vi "ZC_hetong.vi"(0 "action":string, 1 "LabVIEW Web Service Request":refnum<class "Web Request.lvclass"> caption="LabVIEW Web服务请求", 2 "fpbh":string, 3 "gmjg":string, 5 "id":string, 6 "key":string, 7 "name":string, 8 "number":string, 9 "bianhao":string, 10 "shuliang":string, 11 "gysh":string, 12 "gmriqi":string, 13 "bxnx":string, 14 "beizhu":string, 15 "gmzc":string) -> (4 "error":errorcluster)   [LabVIEW 2017]
uses:
  <vilib>/wsapi/Web Request.lvclass
panel:
  out "postdata":string caption="post数据"
  out "error out":errorcluster caption="错误输出"
  # "Web服务请求输入接线端用于调用“Web服务”选板的VI。除非不需要访问该选板，否则不要在连线板上删除这个输入接线端。"
  # "添加至连线板的每一个其他输入控件，在URL中对应于一个输入。如需在接线端模式输出（默认设置）下包含显示控件，则该显示控件必须与连线板相连。"
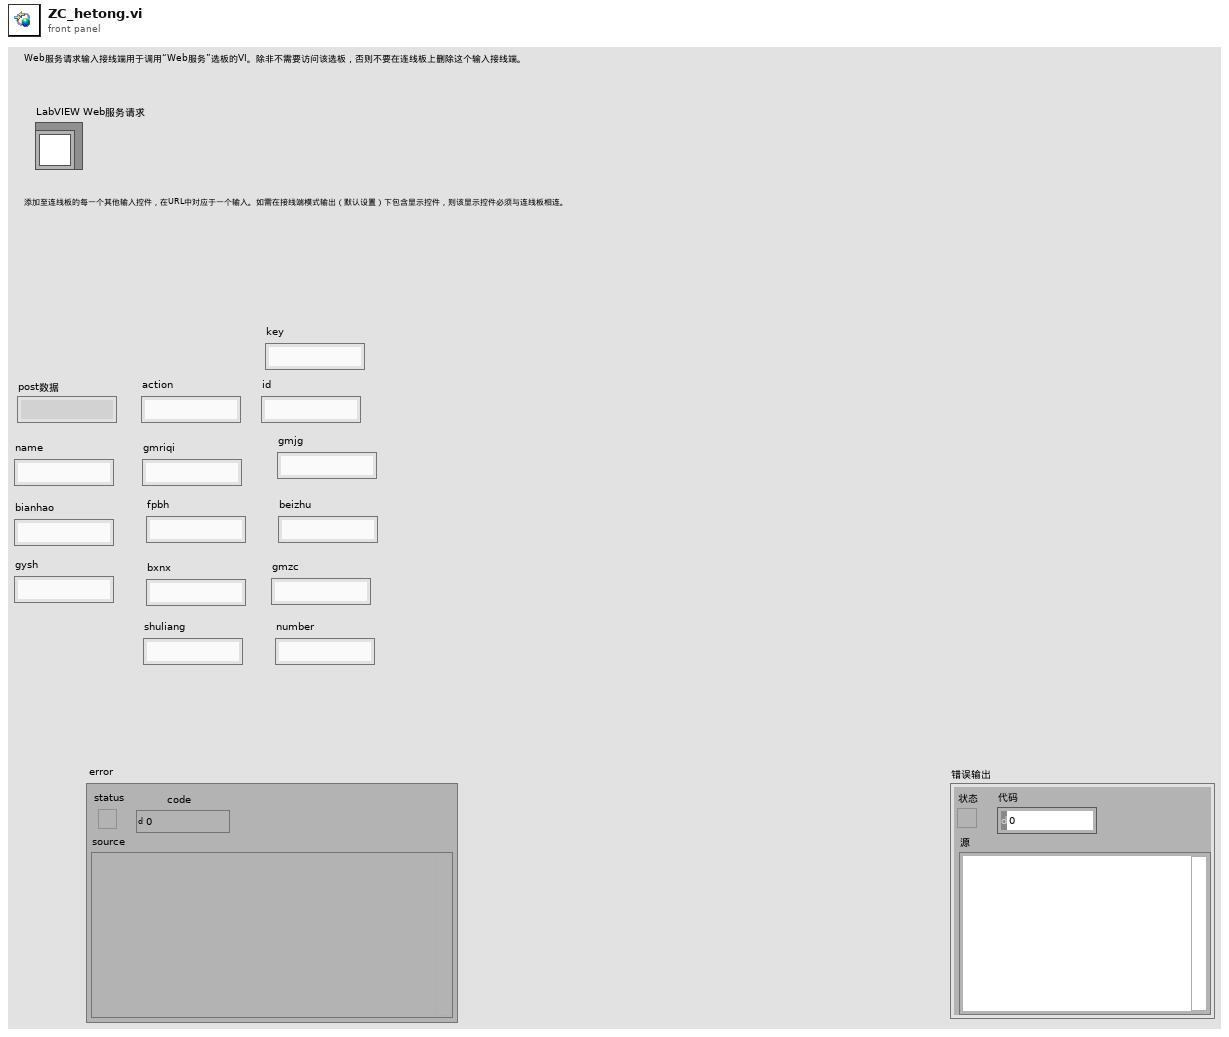
[diagram p1: front panel]
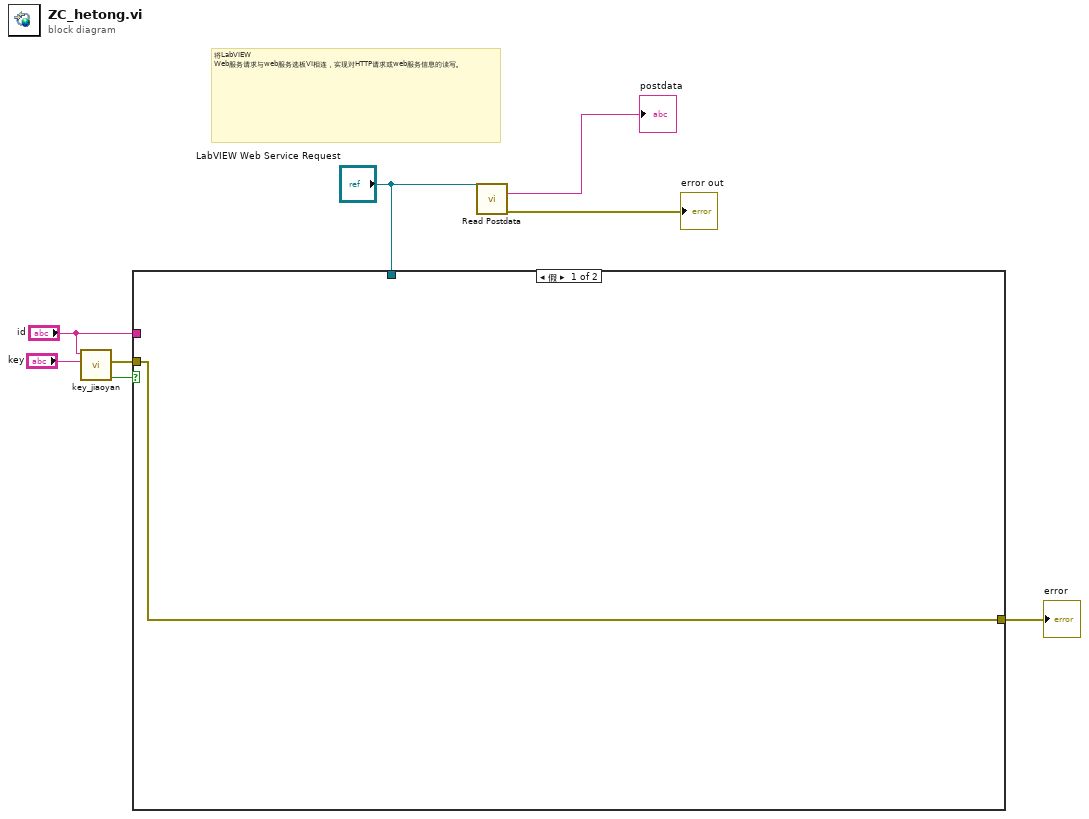
[diagram p0: block diagram]
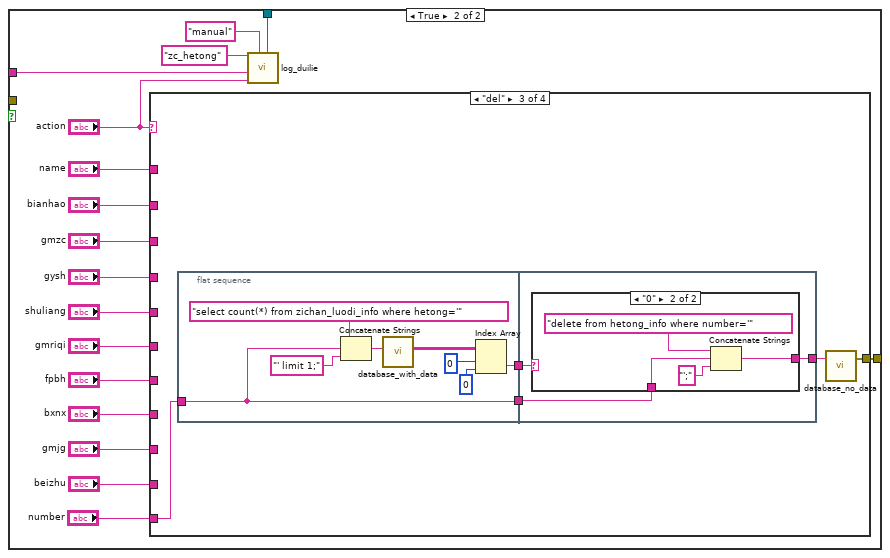
[diagram p2: hidden frame]
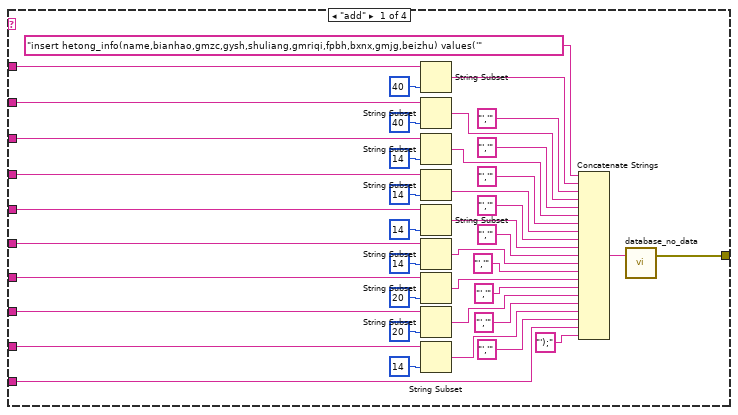
[diagram p3: hidden frame]
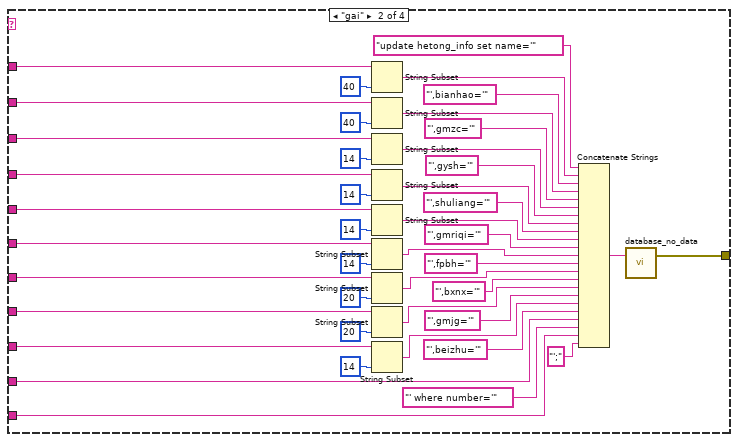
[diagram p4: hidden frame]
diagram:
  # "将LabVIEW Web服务请求与web服务选板VI相连，实现对HTTP请求或web服务信息的读写。"
  n1 = call "key_jiaoyan.vi"("key_client"="key", "gonghao"="id") -> ("jy"=w2:bool, "error"=w1:errorcluster)  [unwired: 8 in]
  n2 = case shown="假" w2 {
    tunnel: [w9 w15] -> w7
    tunnel: "LabVIEW Web Service Request" -> [_ w12]
    tunnel: "id" -> [_ w10]
    tunnel: w1 -> [w9 _]
    frame False {
    }
    frame True {
      n3 = case shown="\"del\"" "action" {
        tunnel: [w37 w85 w111 _] -> w15
        tunnel: "shuliang" -> [w36 w84 _ _]
        tunnel: "gmzc" -> [w35 w83 _ _]
        tunnel: "gmjg" -> [w34 w82 _ _]
        tunnel: "beizhu" -> [w33 w81 _ _]
        tunnel: "bxnx" -> [w32 w80 _ _]
        tunnel: "fpbh" -> [w31 w79 _ _]
        tunnel: "gmriqi" -> [w30 w78 _ _]
        tunnel: "gysh" -> [w29 w77 _ _]
        tunnel: "bianhao" -> [w28 w76 _ _]
        tunnel: "name" -> [w27 w75 _ _]
        tunnel: "number" -> [_ w70 w112 _]
        frame "add" {
          n4 = String Subset(string=w27, length (rest)=40 ("长度（剩余）")) -> (substring=w63:string)  [unwired: 1 in]
          n5 = String Subset(string=w28, length (rest)=40 ("长度（剩余）")) -> (substring=w61:string)  [unwired: 1 in]
          n6 = String Subset(string=w35, length (rest)=14 ("长度（剩余）")) -> (substring=w43:string)  [unwired: 1 in]
          n7 = String Subset(string=w29, length (rest)=14 ("长度（剩余）")) -> (substring=w59:string)  [unwired: 1 in]
          n8 = String Subset(string=w36, length (rest)=14 ("长度（剩余）")) -> (substring=w39:string)  [unwired: 1 in]
          n9 = String Subset(string=w30, length (rest)=14 ("长度（剩余）")) -> (substring=w57:string)  [unwired: 1 in]
          n10 = String Subset(string=w31, length (rest)=20 ("长度（剩余）")) -> (substring=w52:string)  [unwired: 1 in]
          n11 = String Subset(string=w32, length (rest)=20 ("长度（剩余）")) -> (substring=w49:string)  [unwired: 1 in]
          n12 = String Subset(string=w34, length (rest)=14 ("长度（剩余）")) -> (substring=w46:string)  [unwired: 1 in]
          n13 = Concatenate Strings("insert hetong_info(name,bianhao,gmzc,gysh,shuliang,gmriqi,fpbh,bxnx,gmjg,beizhu) values('" ("格式字符串"), w63, "','" ("字符串"), w61, "','" ("字符串"), w43, "','" ("字符串"), w59, "','" ("字符串"), w39, "','" ("字符串"), w57, "','" ("字符串"), w52, "','" ("字符串"), w49, "','" ("字符串"), w46, "','" ("字符串"), w33, "');" ("字符串")) -> (w38:string)
          n14 = call "database_no_data.vi"("input"=w38) -> ("error"=w37:errorcluster)  [unwired: 2 in]
        }
        frame "gai" {
          n15 = String Subset(string=w75, length (rest)=40 ("长度（剩余）")) -> (substring=w106:string)  [unwired: 1 in]
          n16 = String Subset(string=w76, length (rest)=40 ("长度（剩余）")) -> (substring=w104:string)  [unwired: 1 in]
          n17 = String Subset(string=w83, length (rest)=14 ("长度（剩余）")) -> (substring=w90:string)  [unwired: 1 in]
          n18 = String Subset(string=w77, length (rest)=14 ("长度（剩余）")) -> (substring=w73:string)  [unwired: 1 in]
          n19 = String Subset(string=w84, length (rest)=14 ("长度（剩余）")) -> (substring=w72:string)  [unwired: 1 in]
          n20 = String Subset(string=w78, length (rest)=14 ("长度（剩余）")) -> (substring=w101:string)  [unwired: 1 in]
          n21 = String Subset(string=w79, length (rest)=20 ("长度（剩余）")) -> (substring=w68:string)  [unwired: 1 in]
          n22 = String Subset(string=w80, length (rest)=20 ("长度（剩余）")) -> (substring=w74:string)  [unwired: 1 in]
          n23 = String Subset(string=w82, length (rest)=14 ("长度（剩余）")) -> (substring=w93:string)  [unwired: 1 in]
          n24 = Concatenate Strings("update hetong_info set name='" ("格式字符串"), w106, "',bianhao='" ("字符串"), w104, "',gmzc='" ("字符串"), w90, "',gysh='" ("字符串"), w73, "',shuliang='" ("字符串"), w72, "',gmriqi='" ("字符串"), w101, "',fpbh='" ("字符串"), w68, "',bxnx='" ("字符串"), w74, "',gmjg='" ("字符串"), w93, "',beizhu='" ("字符串"), w81, "' where number='" ("字符串"), w70, "';" ("字符串")) -> (w86:string)
          n25 = call "database_no_data.vi"("input"=w86) -> ("error"=w85:errorcluster)  [unwired: 2 in]
        }
        frame "del" {
          n26 = flat-sequence {
            tunnel: w112 -> [w121]
            tunnel: [w121] -> w115
            tunnel: [w116] -> w114
            tunnel: [w126] -> w113
            tunnel: w115 -> [w125]
            tunnel: w114 -> [w124]
            frame #0 {
              n27 = Concatenate Strings("select count(*) from zichan_luodi_info where hetong='" ("格式字符串"), w121, "' limit 1;" ("字符串")) -> (w120:string)
              n28 = call "database_with_data.vi"("input"=w120) -> ("Data"=w117:string[][])  [unwired: 9 in, 1 out]
              n29 = Index Array(array=w117, index (row)=0 ("索引 (行)"), index (col)=0 ("禁用的索引 (列)")) -> (element=w116:string)
            }
            frame #1 {
              n30 = case shown="\"0\"" w124 {
                tunnel: [_ w128] -> w126
                tunnel: w125 -> [_ w127]
                frame "假", Default {
                }
                frame "0" {
                  n31 = Concatenate Strings("delete from hetong_info where number='" ("格式字符串"), w127, "';" ("字符串")) -> (w128:string)
                }
              }
            }
          }
          n32 = call "database_no_data.vi"("input"=w113) -> ("error"=w111:errorcluster)  [unwired: 2 in]
        }
        frame Default {
        }
      }
      n33 = call "log_duilie.vi"("LabVIEW Web Service Request"=w12, "type"="manual", "action"="action", "user"=w10, "yw"="zc_hetong") -> ()  [unwired: 7 in]
    }
  }
  "error" <- w7
  n34 = call <vilib>:"Read Postdata.vi"("LabVIEW Web Service Request"="LabVIEW Web Service Request") -> ("postdata"=→"postdata":string, "error out"=→"error out":errorcluster)  [unwired: 12 in, 1 out]
